vi "FormCalibra7.vi"() -> ()   [LabVIEW 2014]
uses:
  testMachine.ctl
  mainMachine.ctl
  <vilib>/Analysis/baseanly.llb/Mean (DBL).vi
  <vilib>/express/express shared/transition.llb/Dynamic To Waveform Array.vi
  <vilib>/express/express signal manip/GetorSetDDTAttributes/Set DDT Attributes/SetT0.vi
  <vilib>/express/express shared/transition.llb/Waveform Array To Dynamic.vi
  <vilib>/measure/mamon.llb/Trigger Detection for 1 Channel.vi
  <vilib>/express/express signal manip/GetorSetDDTAttributes/Set DDT Attributes/Set DDT Properties.xnode
  <vilib>/Analysis/NI_AALBase.lvlib
  <resource>/objmgr/daqmx.rc
  <vilib>/measure/NI_MAPro.lvlib
panel:
  out "editDistance":dbl caption="Distancia (m)" format="%#_4f"
  in  "Lower level":dbl
  in  "hysteresis":dbl format="%.2p"
  in  "level":dbl format="%.2p"
  out "rpm":bool
  out "deviceName":tag
  out "editTotalWaitLimit":u8
  out "editCountWaitLimit":u8
  out "ledWaitState":bool caption="Wait State"
  out "sliderWaitUpperTime":u8(slide) max=50 scale=0.0..30.0
  out "slideWaitLowerTime":u8(slide) max=30 scale=0.0..1.0
  out "slideWaitTime":u8(slide) scale=0.0..150.0
  out "labelTestTime":string caption="Tempo total de ensaio"
  in  "buttonAcquisition":bool
  in  "editSetWaitTime":u8 caption="Tempo entre ciclos (s)" step=1 format="%0d"
  in  "stop":bool
  out "error out":errorcluster
  out "ledAcquireState":bool caption="Acquire State"
  out "editTotalLowerLimit":u8
  out "editCountLowerLimit":u8
  out "editTotalUpperLimit":u8
  out "editCountUpperLimit":u8
  out "ledEnsaio 3":bool
  out "ledBrakeState":bool caption="Brake State"
  out "ledExitState":bool caption="Exit State"
  out "ledMotorState":bool caption="Motor State"
  out "ledInit2State":bool caption="Init State"
  out "ledBlockState":bool caption="Block State"
  out "ledRunningState":bool caption="Running State"
  out "ledReadyState":bool caption="Ready State"
  out "ledInitState":bool caption="Init State"
  out "mainMachine":T1
  out "testMachine":T2=enum."finish"
  in  "editSetPathToFile":path
  in  "buttonStop":bool
  in  "buttonStart":bool
  out "graphForce":dynamicdata(graph)
  in  "editOffsetForce":dbl caption="Tara" min=0.0 max=100.0 step=0.1
  in  "editSetForce":dbl caption="Fator de conversão"
  out "editForce":dbl caption="Força (Kgf)" format="%#_4f"
  out "graphSpeed":dynamicdata(graph)
  in  "editSetSpeed":dbl caption="Fator de conversão"
  out "editSpeed":dbl caption="Velocidade (km/h)" format="%#_4f"
  out "editEngineSpeed":dbl caption="Rotação (RPM)" format="%#_4f"
  in  "buttonMotor":bool
  in  "buttonBrake":bool
  in  "editSetWaitLowerTime":u8 caption="Tempo de espera (s)"
  in  "editSetWaitUpperTime":u8=3 caption="Tempo de espera (s)"
  in  "editSetNumberOfCycles":u16 caption="Número de ciclos" max=999 step=1 format="%0d"
  in  "editSetLowerLimit":u32 caption="Limite inferior (km/h)"
  in  "editSetUpperLimit":u32 caption="Limite superior (km/h)"
  out "editTempB":dbl caption="Temperatura B (ºC)"
  out "editTempA":dbl caption="Temperatura A (ºC)"
  in  "editSetTempRef":dbl caption="Offset referência" step=0.01 format="%#_2f"
  out "editTempRef":dbl caption="Referência (ºC)"
  out "ledMotor":bool
  out "ledBrake":bool
  out "ledEnsaio":bool
  out "labelTotalCycle":string
  out "labelCurrentCycle":string
  out "labelSystemTitle":string
  in  "editCurrCycleCtr":u32
  in  "velocidade 2":u32
  out "velocidade":u32
  # "Bancada de Frenagem - Ensaio"
  # "Ensaio"
  # "Temperatura"
  # "Rotação"
  # "Célula de Carga"
  # "Configurações do ensaio"
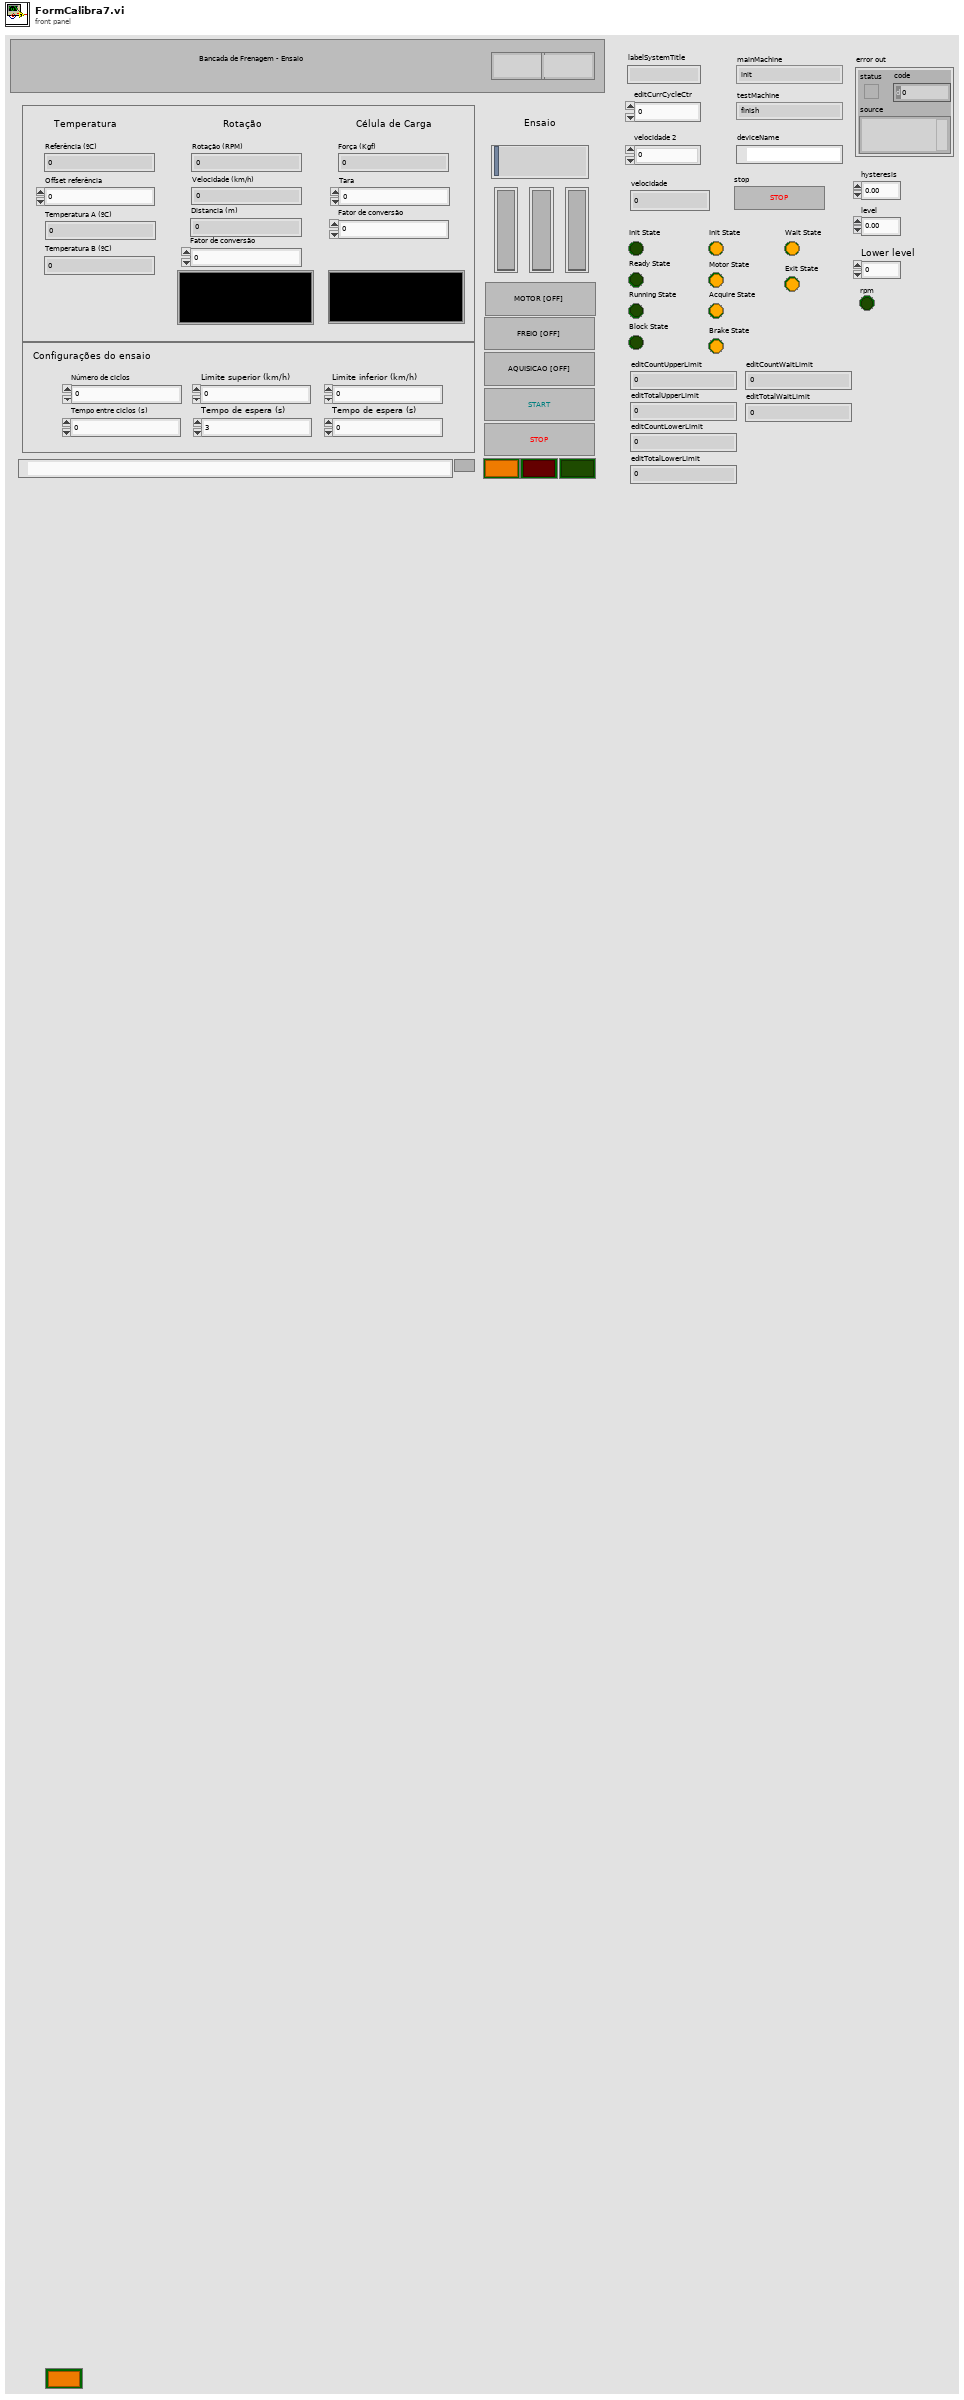
[diagram p1: front panel]
types:
  T1 = typedef "mainMachine.ctl" = enum16{"init", "ready", "running", "blocked", "finish"}
  T2 = typedef "testMachine.ctl" = enum16{"init", "motor", "motor acquire", "brake", "brake acquire", "wait ", "finish", "exit"}
  T3 = enum8{"Enabled", "Disabled", "Disabled and Grayed Out"}
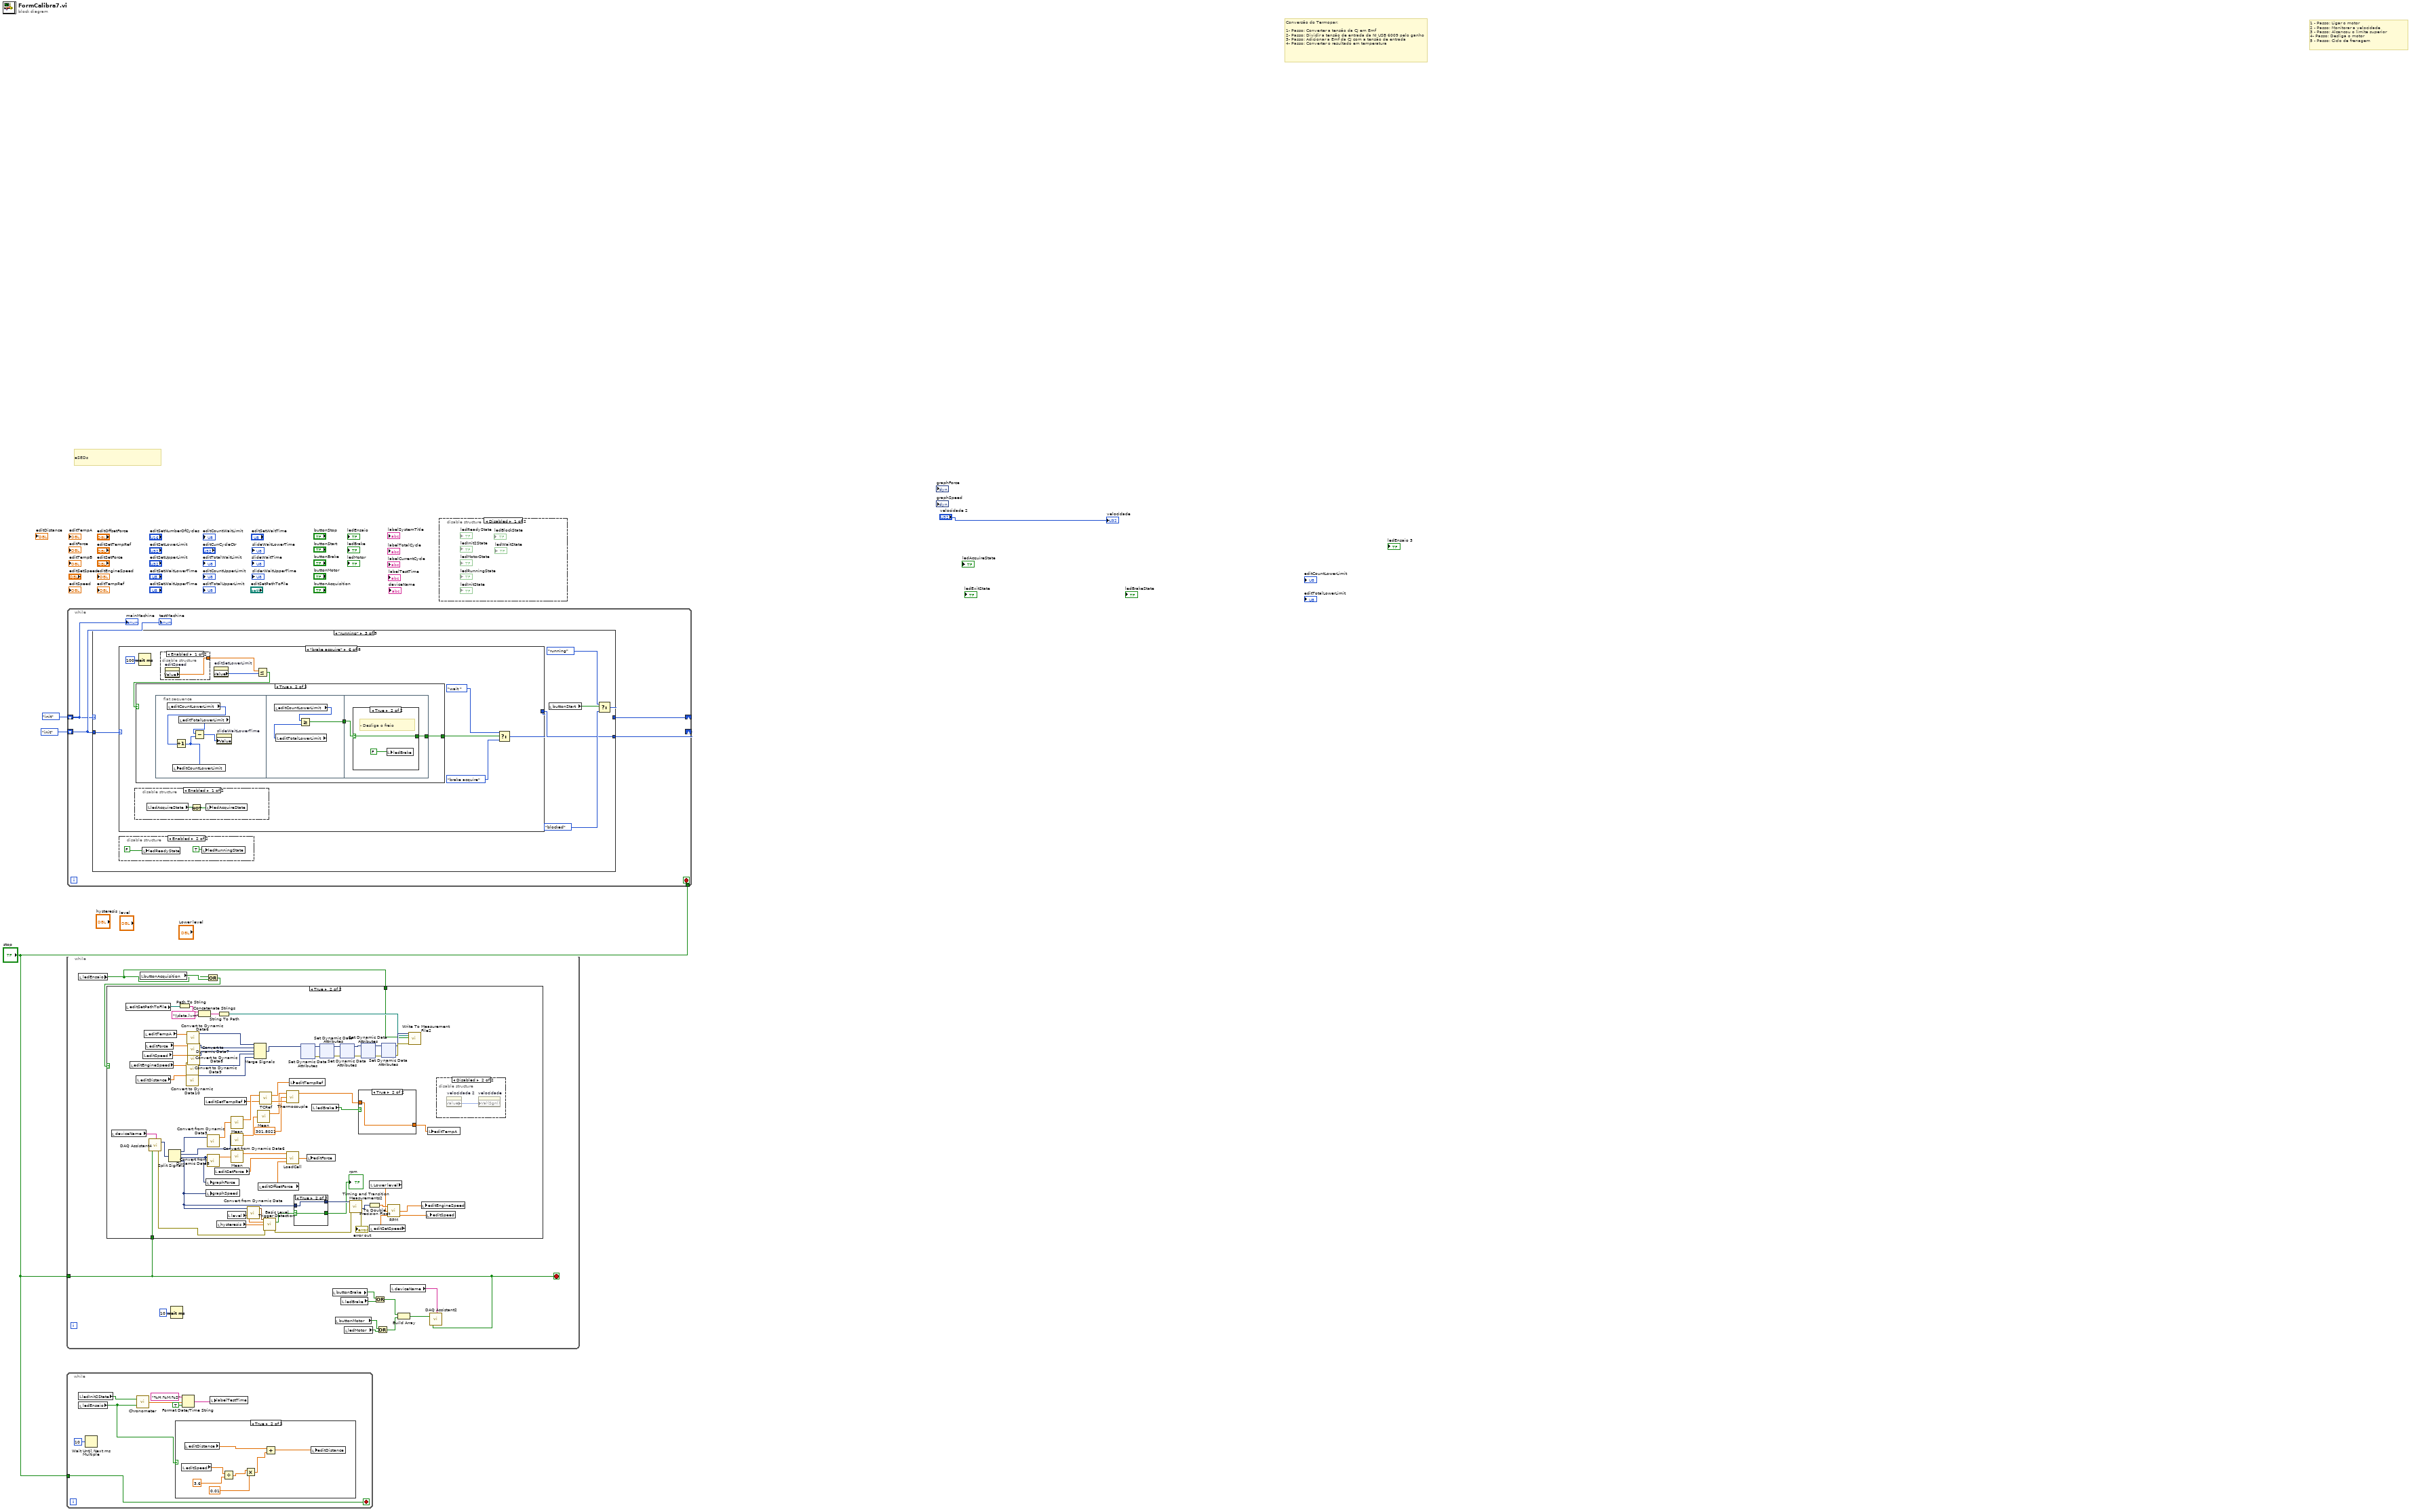
[diagram p0: block diagram]
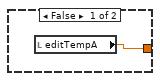
[diagram p5: hidden frame]
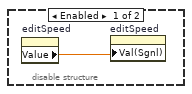
[diagram p7: hidden frame]
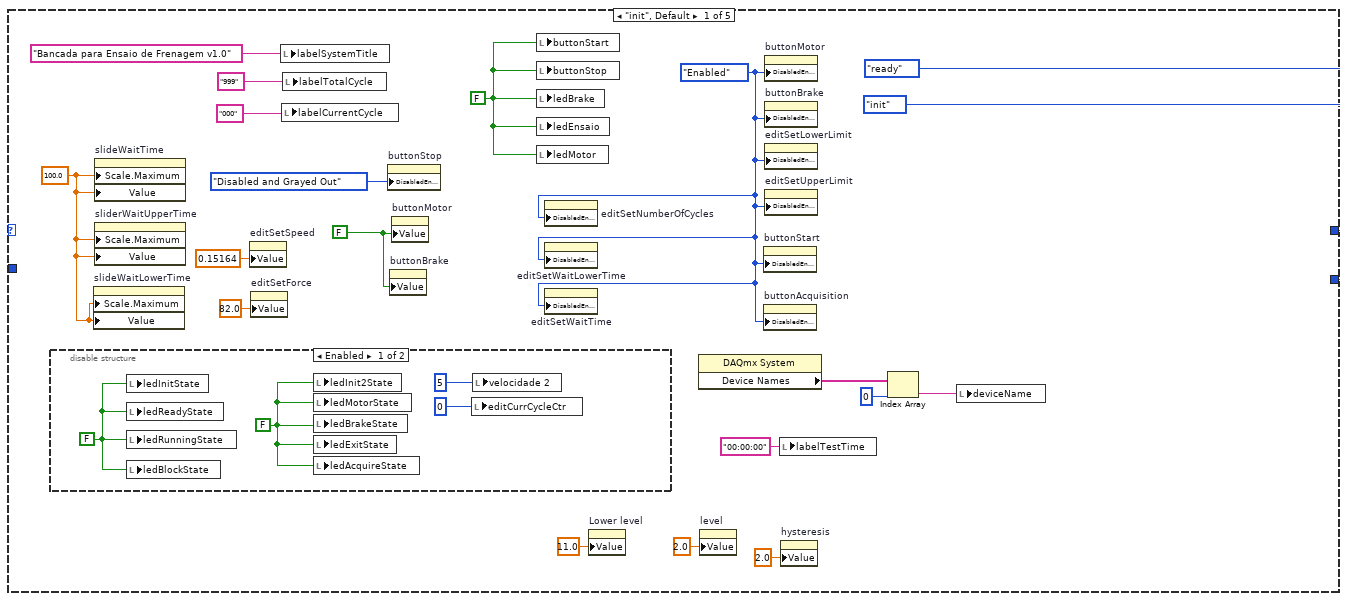
[diagram p8: hidden frame]
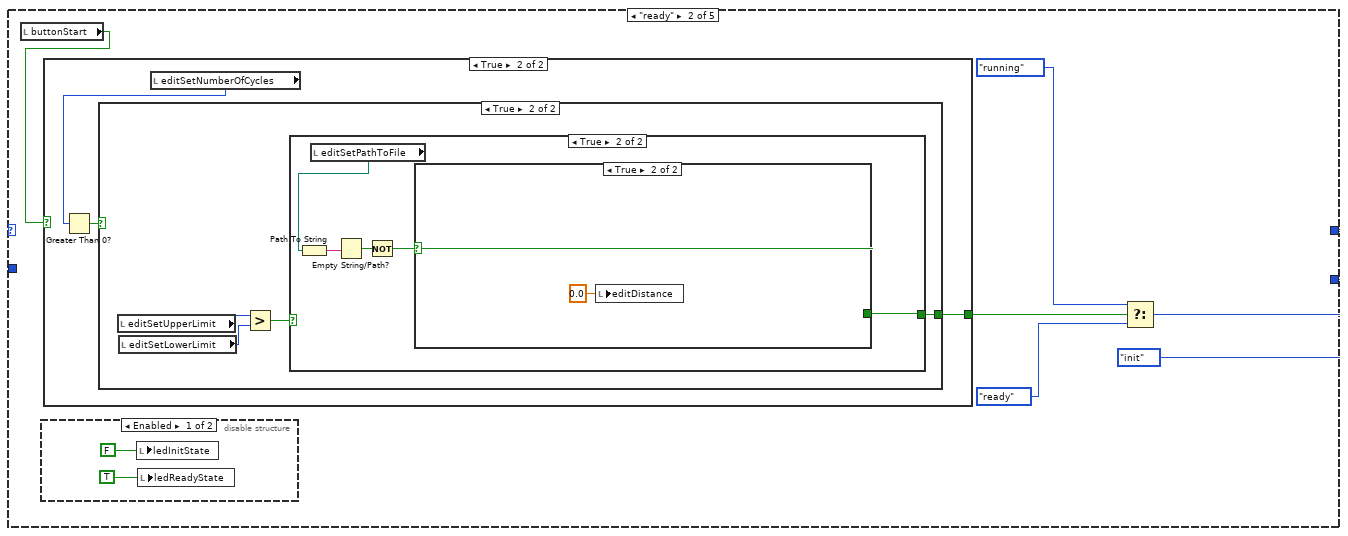
[diagram p10: hidden frame]
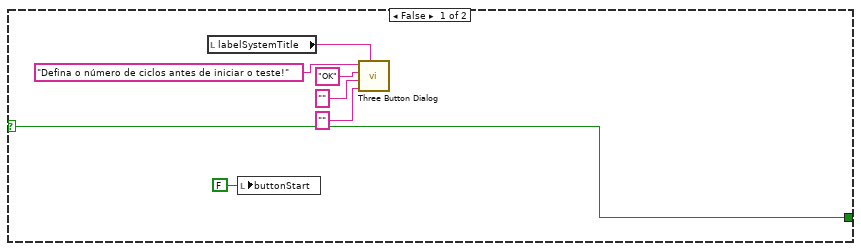
[diagram p13: hidden frame]
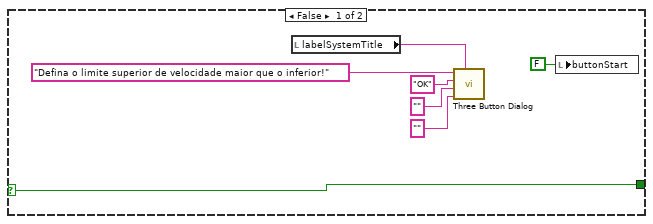
[diagram p14: hidden frame]
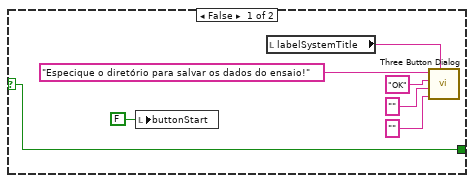
[diagram p15: hidden frame]
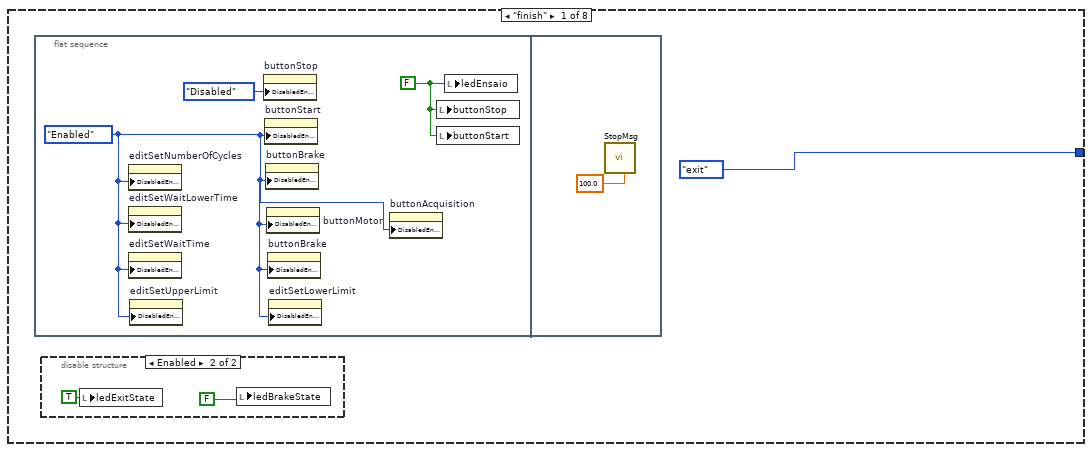
[diagram p17: hidden frame]
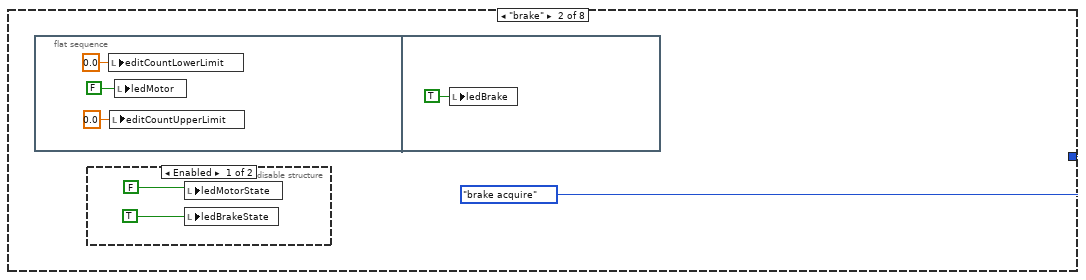
[diagram p19: hidden frame]
diagram:
  # "eSEDs"
  # "1 - Passo: Ligar o motor\n2 - Passo: Monitorar a velocidade\n3 - Passo: Alcancou o limite superior\n4- Passo: Desliga o motor\n5 - Passo: Ciclo de frenagem"
  # "Conversão do Termopar:\n\n1- Passo: Converter a tensão da CJ em Emf\n2- Passo: Dividir a tensão de entrada da NI USB 6009 pelo ganho\n3- Passo: Adicionar a Emf da CJ com a tensão de entrada\n4- Passo: Converter o resultado em temperatura"
  n1 = while {
    tunnel: "stop" -> [w12]
    stop <- w12 stop-if-true
    n2 = local read "ledInit2State"() -> (w7:bool)
    n3 = local read "ledEnsaio"() -> (w5:bool)
    n4 = Wait Until Next ms Multiple(millisecond multiple=u32 10) -> ()  [unwired: 1 out]
    n5 = call "Chronometer.vi"("start"=w5, "reset"=w7) -> ("Time"=w11:dbl)
    n6 = case shown="True" w5 {
      frame False {
      }
      frame True {
        n7 = local read "editSpeed"() -> (w17:dbl)
        n8 = local read "editDistance"() -> (w19:dbl)
        n9 = Divide(x=w17, y=3.6) -> (x/y=w15:dbl)
        n10 = Multiply(x=w15, y=0.01) -> (x*y=w14:dbl)
        n11 = Add(x=w19, y=w14) -> (x+y=w13:dbl)
        n12 = local write "editDistance"(w13) -> ()
      }
    }
    n13 = Format Date/Time String(time format string (%c)="%H:%M:%S", seconds (now)=w11, UTC format=TRUE) -> (date/time string=w8:string)
    n14 = local write "labelTestTime"(w8) -> ()
  }
  n15 = while {
    tunnel: "stop" -> [w25]
    stop <- w25 stop-if-true
    n16 = local read "ledEnsaio"() -> (w22:bool)
    n17 = local read "buttonAcquisition"() -> (w24:bool)
    n18 = Wait (ms)(milliseconds to wait=u32 10) -> ()  [unwired: 1 out]
    n19 = Or(x=w22, y=w24) -> (x .or. y?=w23:bool)
    n20 = case shown="True" w23 {
      tunnel: w25 -> [_ w57]
      tunnel: w22 -> [_ w56]
      frame False {
      }
      frame True {
        n21 = local read "deviceName"() -> (w55:tag)
        n22 = local read "editSetPathToFile"() -> (w77:path)
        n23 = local read "editEngineSpeed"() -> (w39:dbl)
        n24 = local read "editDistance"() -> (w40:dbl)
        n25 = local read "editSpeed"() -> (w37:dbl)
        n26 = local read "editTempA"() -> (w89:dbl)
        n27 = local read "editForce"() -> (w38:dbl)
        n28 = call "DAQ Assistant4"("stop (F)"=w57, "device name"=w55) -> ("data"=w59:dynamicdata, "error out"=w54:errorcluster)  [unwired: 14 in, 2 out]
        n29 = Split Signals(w59) -> (w36:dynamicdata, w35:dynamicdata, w34:dynamicdata, w33:dynamicdata)  [unwired: 4 in]
        n30 = Path To String(path=w77) -> (string=w76:string)
        n31 = call "Convert to Dynamic Data9"("Double"=w39) -> ("Dynamic Data Type"=w93:dynamicdata)  [unwired: 3 in]
        n32 = call "Convert to Dynamic Data10"("Double"=w40) -> ("Dynamic Data Type"=w94:dynamicdata)  [unwired: 3 in]
        n33 = call "Convert to Dynamic Data6"("Double"=w89) -> ("Dynamic Data Type"=w90:dynamicdata)  [unwired: 3 in]
        n34 = call "Convert to Dynamic Data7"("Double"=w38) -> ("Dynamic Data Type"=w91:dynamicdata)  [unwired: 3 in]
        n35 = call "Convert to Dynamic Data8"("Double"=w37) -> ("Dynamic Data Type"=w92:dynamicdata)  [unwired: 3 in]
        n36 = Concatenate Strings(w76, "\\data.lvm" ("string")) -> (w79:string)
        n37 = local read "editSetTempRef"() -> (w61:dbl)
        n38 = local write "graphForce"(w34) -> ()
        n39 = local write "graphSpeed"(w33) -> ()
        n40 = call "Convert from Dynamic Data5"("Dynamic Data Type"=w36) -> ("Array"=w74:dbl[])  [unwired: 3 in]
        n41 = call "Convert from Dynamic Data8"("Dynamic Data Type"=w34) -> ("Array"=w63:dbl[])  [unwired: 3 in]
        n42 = local read "editSetForce"() -> (w72:dbl)
        n43 = local read "hysteresis"() -> (w46:dbl)
        n44 = String To Path(string=w79) -> (path=w80:path)
        n45 = local read "level"() -> (w45:dbl)
        n46 = call-poly <vilib>:"Mean.vi"("X"=w74) -> ("mean"=w75:dbl)  [unwired: 1 out]
        n47 = call "Convert from Dynamic Data6"("Dynamic Data Type"=w35) -> ("Array"=w62:dbl[])  [unwired: 3 in]
        n48 = call-poly <vilib>:"Mean.vi"("X"=w63) -> ("mean"=w67:dbl)  [unwired: 1 out]
        n49 = call "Convert from Dynamic Data"("Dynamic Data Type"=w33) -> ("Waveform"=w51:waveform(dbl))  [unwired: 3 in]
        n50 = Merge Signals(w90, w91, w92, w93, w94) -> (w95:dynamicdata)
        n51 = call-poly <vilib>:"Mean.vi"("X"=w62) -> ("mean"=w64:dbl)  [unwired: 1 out]
        n52 = local read "editOffsetForce"() -> (w73:dbl)
        n53 = call "TCRef.vi"("offset"=w61, "data"=w75) -> ("emf(mV)"=w66:dbl, "temp (degC)"=w60:dbl)
        n54 = call-poly <vilib>:"Basic Level Trigger Detection.vi"("signal in"=w51, "level"=w45, "hysteresis"=w46, "error in (no error)"=w54) -> ("trigger detected?"=w50:bool, "error out"=w53:errorcluster)  [unwired: 9 in, 1 out]
        n55 = call "Thermocouple.vi"("cj(mV)"=w66, "factor"=301.8021, "data"=w64) -> ("temp(degC)"=w42:dbl)  [unwired: 2 out]
        n56 = call "LoadCell.vi"("tara"=w73, "factor"=w72, "data"=w67) -> ("force (Kgf)"=w69:dbl)
        n57 = local write "editTempRef"(w60) -> ()
        n58 = case shown="True" w50 {
          selector: w50 -> [w100 w101]
          tunnel: w33 -> [_ w102]
          tunnel: [_ w102] -> w52
          tunnel: [w100 w101] -> w49
          frame False {
          }
          frame True {
          }
        }
        "rpm" <- w49
        n59 = xnode ("Set Dynamic Data Attributes")("Signals In"=w95) -> ("Signals Out"=w81:dynamicdata, "error out"=w83:errorcluster)  [unwired: 4 in]
        n60 = local write "editForce"(w69) -> ()
        n61 = local read "ledBrake"() -> (w43:bool)
        n62 = xnode ("Set Dynamic Data Attributes")("Signals In"=w81, "error in"=w83) -> ("Signals Out"=w82:dynamicdata, "error out"=w84:errorcluster)  [unwired: 3 in]
        n63 = xnode ("Set Dynamic Data Attributes")("Signals In"=w82, "error in"=w84) -> ("Signals Out"=w96:dynamicdata, "error out"=w85:errorcluster)  [unwired: 3 in]
        n64 = call "Timing and Transition Measurements2"("error in (no error)"=w53, "Signals"=w52) -> ("error out"=→"error out":errorcluster, "Frequency"=w48:dynamicdata)  [unwired: 8 in]
        n65 = case shown="True" w43 {
          tunnel: w42 -> [_ w99]
          tunnel: [w98 w99] -> w41
          frame False {
            n66 = local read "editTempA"() -> (w98:dbl)
          }
          frame True {
          }
        }
        n67 = xnode ("Set Dynamic Data Attributes")("Signals In"=w96, "error in"=w85) -> ("Signals Out"=w97:dynamicdata, "error out"=w86:errorcluster)  [unwired: 3 in]
        n68 = To Double Precision Float(number=w48) -> (double precision float=w47:dbl)
        n69 = local read "Lower level"() -> (w44:dbl)
        n70 = local read "editSetSpeed"() -> (w68:dbl)
        n71 = xnode ("Set Dynamic Data Attributes")("Signals In"=w97, "error in"=w86) -> ("Signals Out"=w87:dynamicdata, "error out"=w88:errorcluster)  [unwired: 3 in]
        n72 = call "RPM.vi"("factor"=w68, "Lower level"=w44, "data"=w47) -> ("km/h"=w71:dbl, "RPM"=w70:dbl)  [unwired: 1 out]
        n73 = call "Write To Measurement File2"("Signals"=w87, "Enable"=w56, "error in (no error)"=w88, "Filename"=w80) -> ()  [unwired: 13 in, 3 out]
        n74 = local write "editEngineSpeed"(w70) -> ()
        n75 = local write "editSpeed"(w71) -> ()
        n76 = local write "editTempA"(w41) -> ()
        n77 = disable-structure shown="Disabled" {
          frame Enabled {
            n78 = property on="editSpeed" class="DigNum (strict)"() -> ("Value"=w103:dbl)  [unwired: 2 in, 2 out]
            n79 = property on="editSpeed" class="DigNum (strict)"("Val(Sgnl)"=w103) -> ()  [unwired: 2 in, 2 out]
          }
          frame Disabled {
            n80 = property on="velocidade 2" class="DigNum (strict)"() -> ("Value"=w104:u32)  [unwired: 2 in, 2 out]
            n81 = property on="velocidade" class="DigNum (strict)"("Val(Sgnl)"=w104) -> ()  [unwired: 2 in, 2 out]
          }
        }
      }
    }
    n82 = local read "buttonBrake"() -> (w29:bool)
    n83 = local read "buttonMotor"() -> (w27:bool)
    n84 = local read "ledBrake"() -> (w31:bool)
    n85 = local read "ledMotor"() -> (w28:bool)
    n86 = Or(x=w29, y=w31) -> (x .or. y?=w30:bool)
    n87 = Or(x=w27, y=w28) -> (x .or. y?=w26:bool)
    n88 = local read "deviceName"() -> (w20:tag)
    n89 = Build Array(w30, w26) -> (w32:bool[])
    n90 = call "DAQ Assistant2"("data"=w32, "stop (T)"=w25, "device name"=w20) -> ()  [unwired: 15 in, 2 out]
  }
  n91 = while {
    shift-right: [w199] -> _
    shift-left: mainMachine."init" ("mainMachine") -> [w196]
    shift-right: [w198] -> _
    shift-left: testMachine."init" ("testMachine") -> [w197]
    tunnel: "stop" -> [w195]
    stop <- w195 stop-if-true
    n92 = case shown="\"running\"" w196 {
      tunnel: [mainMachine."ready" ("mainMachine") w223 w269 w409 mainMachine."finish" ("mainMachine")] -> w199
      tunnel: [testMachine."init" ("testMachine") testMachine."init" ("testMachine") w268 testMachine."init" ("testMachine") testMachine."init" ("testMachine")] -> w198
      tunnel: w197 -> [_ _ w267 _ _]
      frame "init", Default {
        w209 = 100.0 ("Scale.Range:Maximum")
        w210 = T3."Enabled" ("Disabled")
        w211 = FALSE ("buttonMotor")
        w217 = FALSE ("motor")
        n93 = disable-structure shown="Enabled" {
          frame Enabled {
            w219 = FALSE
            w220 = FALSE
            n94 = local write "ledInitState"(w220) -> ()
            n95 = local write "ledReadyState"(w220) -> ()
            n96 = local write "ledRunningState"(w220) -> ()
            n97 = local write "ledBlockState"(w220) -> ()
            n98 = local write "ledInit2State"(w219) -> ()
            n99 = local write "ledMotorState"(w219) -> ()
            n100 = local write "ledBrakeState"(w219) -> ()
            n101 = local write "ledExitState"(w219) -> ()
            n102 = local write "ledAcquireState"(w219) -> ()
            n103 = local write "editCurrCycleCtr"(u32 0 ("currentCycleCtr")) -> ()
            n104 = local write "velocidade 2"(u32 5 ("velocidade 2")) -> ()
          }
          frame Disabled {
          }
        }
        n105 = property on="slideWaitLowerTime" class="Slide (strict)"("Scale.Maximum"=w209, "Value"=w209) -> ()  [unwired: 2 in, 2 out]
        n106 = property on="slideWaitTime" class="Slide (strict)"("Scale.Maximum"=w209, "Value"=w209) -> ()  [unwired: 2 in, 2 out]
        n107 = property on="sliderWaitUpperTime" class="Slide (strict)"("Scale.Maximum"=w209, "Value"=w209) -> ()  [unwired: 2 in, 2 out]
        n108 = property on="editSetSpeed" class="DigNum (strict)"("Value"=0.15164 ("editSetSpeed")) -> ()  [unwired: 2 in, 2 out]
        n109 = property on="editSetForce" class="DigNum (strict)"("Value"=82.0 ("editSetForce")) -> ()  [unwired: 2 in, 2 out]
        n110 = local write "labelSystemTitle"("Bancada para Ensaio de Frenagem v1.0" ("systemTitle")) -> ()
        n111 = local write "labelCurrentCycle"("000" ("currentCycle")) -> ()
        n112 = local write "labelTotalCycle"("999" ("totalCycle")) -> ()
        n113 = property on="buttonStop" class="Bool (strict)"("DisabledEnum"=T3."Disabled and Grayed Out" ("Disabled")) -> ()  [unwired: 2 in, 2 out]
        n114 = property on="buttonBrake" class="Bool (strict)"("Value"=w211) -> ()  [unwired: 2 in, 2 out]
        n115 = property on="buttonMotor" class="Bool (strict)"("Value"=w211) -> ()  [unwired: 2 in, 2 out]
        n116 = local write "buttonStart"(w217) -> ()
        n117 = local write "buttonStop"(w217) -> ()
        n118 = local write "ledBrake"(w217) -> ()
        n119 = local write "ledEnsaio"(w217) -> ()
        n120 = local write "ledMotor"(w217) -> ()
        n121 = property on="editSetNumberOfCycles" class="DigNum (strict)"("DisabledEnum"=w210) -> ()  [unwired: 2 in, 2 out]
        n122 = property on="editSetWaitLowerTime" class="DigNum (strict)"("DisabledEnum"=w210) -> ()  [unwired: 2 in, 2 out]
        n123 = property on="editSetWaitTime" class="DigNum (strict)"("DisabledEnum"=w210) -> ()  [unwired: 2 in, 2 out]
        n124 = property on="Lower level" class="DigNum (strict)"("Value"=11.0 ("Lower level")) -> ()  [unwired: 2 in, 2 out]
        n125 = property class="DAQmx System"() -> ("Device Names"=w208:tag[])  [unwired: 2 in, 2 out]
        n126 = property on="level" class="DigNum (strict)"("Value"=2.0 ("level")) -> ()  [unwired: 2 in, 2 out]
        n127 = property on="buttonStart" class="Bool (strict)"("DisabledEnum"=w210) -> ()  [unwired: 2 in, 2 out]
        n128 = property on="buttonAcquisition" class="Bool (strict)"("DisabledEnum"=w210) -> ()  [unwired: 2 in, 2 out]
        n129 = property on="buttonMotor" class="Bool (strict)"("DisabledEnum"=w210) -> ()  [unwired: 2 in, 2 out]
        n130 = property on="buttonBrake" class="Bool (strict)"("DisabledEnum"=w210) -> ()  [unwired: 2 in, 2 out]
        n131 = property on="editSetLowerLimit" class="DigNum (strict)"("DisabledEnum"=w210) -> ()  [unwired: 2 in, 2 out]
        n132 = property on="editSetUpperLimit" class="DigNum (strict)"("DisabledEnum"=w210) -> ()  [unwired: 2 in, 2 out]
        n133 = local write "labelTestTime"("00:00:00" ("labelTestTime")) -> ()
        n134 = property on="hysteresis" class="DigNum (strict)"("Value"=2.0 ("hysteresis")) -> ()  [unwired: 2 in, 2 out]
        n135 = Index Array(array=w208, index=0) -> (element=w206:tag)
        n136 = local write "deviceName"(w206) -> ()
      }
      frame "ready" {
        n137 = local read "buttonStart"() -> (w226:bool)
        n138 = disable-structure shown="Enabled" {
          frame Enabled {
            n139 = local write "ledInitState"(FALSE ("ledReady")) -> ()
            n140 = local write "ledReadyState"(TRUE ("ledReady")) -> ()
          }
          frame Disabled {
          }
        }
        n141 = case shown="True" w226 {
          selector: w226 -> [w231 _]
          tunnel: [w231 w232] -> w225
          frame False {
          }
          frame True {
            n142 = local read "editSetNumberOfCycles"() -> (w233:u16)
            n143 = Greater Than 0?(x=w233) -> (x > 0?=w234:bool)
            n144 = case shown="True" w234 {
              selector: w234 -> [w241 _]
              tunnel: [w241 w242] -> w232
              frame False {
                n145 = local read "labelSystemTitle"() -> (w236:string)
                n146 = local write "buttonStart"(FALSE ("startButton")) -> ()
                n147 = call <vilib>:"Three Button Dialog.vi"("Window Title (\"\")"=w236, "Right Button Text (\"Cancel\")"="" ("Right Button Text (\"Cancel\")"), "Center Button Text (\"No\")"="" ("Center Button Text (\"No\")"), "Left Button Text (\"Yes\")"="OK" ("Left Button Text (\"Yes\")"), "message"="Defina o número de ciclos antes de iniciar o teste!") -> ()  [unwired: 6 in, 1 out]
              }
              frame True {
                n148 = local read "editSetUpperLimit"() -> (w244:u32)
                n149 = local read "editSetLowerLimit"() -> (w243:u32)
                n150 = Greater?(x=w244, y=w243) -> (0:w245:bool)
                n151 = case shown="True" w245 {
                  selector: w245 -> [w252 _]
                  tunnel: [w252 w255] -> w242
                  frame False {
                    n152 = local read "labelSystemTitle"() -> (w247:string)
                    n153 = call <vilib>:"Three Button Dialog.vi"("Window Title (\"\")"=w247, "Right Button Text (\"Cancel\")"="" ("Right Button Text (\"Cancel\")"), "Center Button Text (\"No\")"="" ("Center Button Text (\"No\")"), "Left Button Text (\"Yes\")"="OK" ("Left Button Text (\"Yes\")"), "message"="Defina o limite superior de velocidade maior que o inferior!") -> ()  [unwired: 6 in, 1 out]
                    n154 = local write "buttonStart"(FALSE ("startButton")) -> ()
                  }
                  frame True {
                    n155 = local read "editSetPathToFile"() -> (w257:path)
                    n156 = Path To String(path=w257) -> (string=w256:string)
                    n157 = Empty String/Path?(string/path=w256) -> (empty?=w254:bool)
                    n158 = Not(x=w254) -> (.not. x?=w253:bool)
                    n159 = case shown="True" w253 {
                      selector: w253 -> [w264 w266]
                      tunnel: [w264 w266] -> w255
                      frame False {
                        n160 = local write "buttonStart"(FALSE ("startButton")) -> ()
                        n161 = local read "labelSystemTitle"() -> (w259:string)
                        n162 = call <vilib>:"Three Button Dialog.vi"("Window Title (\"\")"=w259, "Right Button Text (\"Cancel\")"="" ("Right Button Text (\"Cancel\")"), "Center Button Text (\"No\")"="" ("Center Button Text (\"No\")"), "Left Button Text (\"Yes\")"="OK" ("Left Button Text (\"Yes\")"), "message"="Especique o diretório para salvar os dados do ensaio!") -> ()  [unwired: 6 in, 1 out]
                      }
                      frame True {
                        n163 = local write "editDistance"(0.0 ("editDistance")) -> ()
                      }
                    }
                  }
                }
              }
            }
          }
        }
        n164 = Select(t=mainMachine."running" ("mainMachine"), s=w225, f=mainMachine."ready" ("mainMachine")) -> (s? t:f=w223:T1)
      }
      frame "running" {
        n165 = case shown="\"brake acquire\"" w267 {
          tunnel: [testMachine."exit" ("testMachine") testMachine."brake acquire" ("testMachine") testMachine."motor acquire" ("testMachine") testMachine."motor" ("testMachine") w339 w359 testMachine."exit" ("testMachine") w392] -> w268
          frame "finish" {
            n166 = flat-sequence {
              frame #0 {
                w279 = FALSE ("ledReady")
                w278 = T3."Enabled" ("Disabled")
                n167 = property on="editSetNumberOfCycles" class="DigNum (strict)"("DisabledEnum"=w278) -> ()  [unwired: 2 in, 2 out]
                n168 = property on="editSetWaitLowerTime" class="DigNum (strict)"("DisabledEnum"=w278) -> ()  [unwired: 2 in, 2 out]
                n169 = property on="editSetWaitTime" class="DigNum (strict)"("DisabledEnum"=w278) -> ()  [unwired: 2 in, 2 out]
                n170 = property on="editSetUpperLimit" class="DigNum (strict)"("DisabledEnum"=w278) -> ()  [unwired: 2 in, 2 out]
                n171 = property on="buttonStop" class="Bool (strict)"("DisabledEnum"=T3."Disabled" ("Disabled")) -> ()  [unwired: 2 in, 2 out]
                n172 = property on="buttonStart" class="Bool (strict)"("DisabledEnum"=w278) -> ()  [unwired: 2 in, 2 out]
                n173 = property on="buttonBrake" class="Bool (strict)"("DisabledEnum"=w278) -> ()  [unwired: 2 in, 2 out]
                n174 = property on="buttonMotor" class="Bool (strict)"("DisabledEnum"=w278) -> ()  [unwired: 2 in, 2 out]
                n175 = property on="buttonBrake" class="Bool (strict)"("DisabledEnum"=w278) -> ()  [unwired: 2 in, 2 out]
                n176 = property on="editSetLowerLimit" class="DigNum (strict)"("DisabledEnum"=w278) -> ()  [unwired: 2 in, 2 out]
                n177 = property on="buttonAcquisition" class="Bool (strict)"("DisabledEnum"=w278) -> ()  [unwired: 2 in, 2 out]
                n178 = local write "buttonStop"(w279) -> ()
                n179 = local write "buttonStart"(w279) -> ()
                n180 = local write "ledEnsaio"(w279) -> ()
              }
              frame #1 {
                n181 = call "StopMsg.vi"("Max Value (100)"=100.0) -> ()  [unwired: 8 in, 2 out]
              }
            }
            n182 = disable-structure shown="Enabled" {
              frame Disabled {
              }
              frame Enabled {
                n183 = local write "ledExitState"(TRUE ("ledReady")) -> ()
                n184 = local write "ledBrakeState"(FALSE ("ledReady")) -> ()
              }
            }
          }
          frame "brake" {
            n185 = flat-sequence {
              frame #0 {
                n186 = local write "editCountLowerLimit"(0.0 ("editCountUpperLimit")) -> ()
                n187 = local write "editCountUpperLimit"(0.0 ("editCountUpperLimit")) -> ()
                n188 = local write "ledMotor"(FALSE ("motor")) -> ()
              }
              frame #1 {
                n189 = local write "ledBrake"(TRUE ("freio")) -> ()
              }
            }
            n190 = disable-structure shown="Enabled" {
              frame Enabled {
                n191 = local write "ledMotorState"(FALSE ("ledReady")) -> ()
                n192 = local write "ledBrakeState"(TRUE ("ledReady")) -> ()
              }
              frame Disabled {
              }
            }
          }
          frame "motor" {
            n193 = flat-sequence {
              frame #0 {
                n194 = local read "editCurrCycleCtr"() -> (w294:u32)
                n195 = Increment(x=w294) -> (x+1=w293:u32)
                n196 = local write "editCurrCycleCtr"(w293) -> ()
              }
              frame #1 {
                n197 = local read "editCurrCycleCtr"() -> (w301:u32)
                n198 = local read "editTotalWaitLimit"() -> (w295:u8)
                n199 = local read "editTotalUpperLimit"() -> (w297:u8)
                n200 = local read "editTotalLowerLimit"() -> (w296:u8)
                n201 = local write "editCountLowerLimit"(u8 0 ("editCountLowerLimit")) -> ()
                n202 = local write "editCountWaitLimit"(u8 0 ("editCountWaitLimit")) -> ()
                n203 = local write "editCountUpperLimit"(u8 0 ("editCountUpperLimit")) -> ()
                n204 = Format Into String(format string="%03d", w301) -> (resulting string=w302:string)  [unwired: 2 in, 1 out]
                n205 = property on="sliderWaitUpperTime" class="Slide (strict)"("Value"=w297) -> ()  [unwired: 2 in, 2 out]
                n206 = property on="slideWaitLowerTime" class="Slide (strict)"("Value"=w296) -> ()  [unwired: 2 in, 2 out]
                n207 = property on="slideWaitTime" class="Slide (strict)"("Value"=w295) -> ()  [unwired: 2 in, 2 out]
                n208 = local write "labelCurrentCycle"(w302) -> ()
              }
              frame #2 {
                # "- Liga o motor"
                n209 = local write "ledMotor"(TRUE ("motor")) -> ()
                n210 = property on="buttonStop" class="Bool (strict)"("DisabledEnum"=T3."Enabled" ("Disabled")) -> ()  [unwired: 2 in, 2 out]
                n211 = property on="buttonStart" class="Bool (strict)"("DisabledEnum"=T3."Disabled and Grayed Out" ("Disabled")) -> ()  [unwired: 2 in, 2 out]
              }
            }
            n212 = disable-structure shown="Enabled" {
              frame Enabled {
                n213 = local write "ledInit2State"(FALSE ("ledReady")) -> ()
                n214 = local write "ledBrakeState"(FALSE ("ledReady")) -> ()
                n215 = local write "ledMotorState"(TRUE ("ledReady")) -> ()
              }
              frame Disabled {
              }
            }
          }
          frame "init", Default {
            n216 = stacked-sequence {
              frame #0 {
                w314 = FALSE ("ensaio")
                n217 = property on="buttonBrake" class="Bool (strict)"("Value"=w314) -> ()  [unwired: 2 in, 2 out]
                n218 = local write "ledMotor"(w314) -> ()
                n219 = local write "ledBrake"(w314) -> ()
                n220 = property on="buttonMotor" class="Bool (strict)"("Value"=w314) -> ()  [unwired: 2 in, 2 out]
                n221 = local read "editSetNumberOfCycles"() -> (w321:u16)
                n222 = local read "editSetWaitLowerTime"() -> (w315:u8)
                n223 = local read "editSetWaitUpperTime"() -> (w318:u8)
                n224 = local read "editSetWaitTime"() -> (w309:u8)
                n225 = Multiply(x=w309, y=u32 10) -> (x*y=w310:u32)
                n226 = Multiply(x=w315, y=u32 10) -> (x*y=w313:u32)
                n227 = Format Into String(format string="%03d", w321) -> (resulting string=w322:string)  [unwired: 2 in, 1 out]
                n228 = Multiply(x=w318, y=u32 10) -> (x*y=w312:u32)
                n229 = local write "editTotalLowerLimit"(w313) -> ()
                n230 = local write "editTotalUpperLimit"(w312) -> ()
                n231 = local write "editTotalWaitLimit"(w310) -> ()
                n232 = local write "labelTotalCycle"(w322) -> ()
                n233 = local write "editCurrCycleCtr"(u32 0 ("currentCycleCtr")) -> ()
                n234 = local write "labelCurrentCycle"("000" ("currentCycle")) -> ()
              }
              frame #1 {
                w330 = T3."Disabled" ("Disabled")
                n235 = property on="editSetNumberOfCycles" class="DigNum (strict)"("DisabledEnum"=w330) -> ()  [unwired: 2 in, 2 out]
                n236 = property on="editSetWaitLowerTime" class="DigNum (strict)"("DisabledEnum"=w330) -> ()  [unwired: 2 in, 2 out]
                n237 = property on="editSetWaitTime" class="DigNum (strict)"("DisabledEnum"=w330) -> ()  [unwired: 2 in, 2 out]
                n238 = local read "editTotalUpperLimit"() -> (w333:u8)
                n239 = property on="sliderWaitUpperTime" class="Slide (strict)"("Scale.Maximum"=w333, "Scale.Minimum"=0.0 ("Scale.Range:Minimum"), "Scale.Increment"=1.0 ("Scale.Range:Increment"), "Value"=w333) -> ()  [unwired: 2 in, 2 out]
                n240 = property on="buttonAcquisition" class="Bool (strict)"("DisabledEnum"=w330) -> ()  [unwired: 2 in, 2 out]
                n241 = local read "editTotalLowerLimit"() -> (w327:u8)
                n242 = property on="slideWaitLowerTime" class="Slide (strict)"("Scale.Maximum"=w327, "Scale.Minimum"=0.0 ("Scale.Range:Minimum"), "Scale.Increment"=1.0 ("Scale.Range:Increment"), "Value"=w327) -> ()  [unwired: 2 in, 2 out]
                n243 = local read "editTotalWaitLimit"() -> (w324:u8)
                n244 = property on="slideWaitTime" class="Slide (strict)"("Scale.Maximum"=w324, "Scale.Minimum"=0.0 ("Scale.Range:Minimum"), "Scale.Increment"=1.0 ("Scale.Range:Increment"), "Value"=w324) -> ()  [unwired: 2 in, 2 out]
                n245 = call "StarMsg.vi"("Show"=TRUE, "Max Value (100)"=100.0) -> ()  [unwired: 7 in, 2 out]
                n246 = property on="buttonMotor" class="Bool (strict)"("DisabledEnum"=w330) -> ()  [unwired: 2 in, 2 out]
                n247 = property on="buttonBrake" class="Bool (strict)"("DisabledEnum"=w330) -> ()  [unwired: 2 in, 2 out]
                n248 = property on="editSetLowerLimit" class="DigNum (strict)"("DisabledEnum"=w330) -> ()  [unwired: 2 in, 2 out]
                n249 = property on="editSetUpperLimit" class="DigNum (strict)"("DisabledEnum"=w330) -> ()  [unwired: 2 in, 2 out]
              }
              frame #2 {
                n250 = local write "ledEnsaio"(TRUE ("ensaio")) -> ()
              }
            }
            n251 = disable-structure shown="Enabled" {
              frame Enabled {
                n252 = local write "ledInit2State"(TRUE ("ledReady")) -> ()
              }
              frame Disabled {
              }
            }
          }
          frame "motor acquire" {
            n253 = disable-structure shown="Enabled" {
              frame Enabled {
                n254 = local read "ledAcquireState"() -> (w348:bool)
                n255 = Not(x=w348) -> (.not. x?=w347:bool)
                n256 = local write "ledAcquireState"(w347) -> ()
              }
              frame Disabled {
              }
            }
            n257 = Wait (ms)(milliseconds to wait=u32 100) -> ()  [unwired: 1 out]
            n258 = disable-structure shown="Enabled" {
              disable-tunnel: [w345 w346] -> w338
              frame Enabled {
                n259 = property on="editSpeed" class="DigNum (strict)"() -> ("Value"=w345:dbl)  [unwired: 2 in, 2 out]
              }
              frame Disabled {
                n260 = property on="velocidade" class="DigNum (strict)"() -> ("Value"=w346:u32)  [unwired: 2 in, 2 out]
              }
            }
            n261 = property on="editSetUpperLimit" class="DigNum (strict)"() -> ("Value"=w337:u32)  [unwired: 2 in, 2 out]
            n262 = Greater Or Equal?(x=w338, y=w337) -> (x >= y?=w343:bool)
            n263 = case shown="True" w343 {
              selector: w343 -> [w349 _]
              tunnel: [w349 w350] -> w342
              frame False {
              }
              frame True {
                n264 = flat-sequence {
                  tunnel: [w355] -> w350
                  frame #0 {
                    n265 = local read "editCountUpperLimit"() -> (w353:u8)
                    n266 = Increment(x=w353) -> (x+1=w351:u8)
                    n267 = local write "editCountUpperLimit"(w351) -> ()
                    n268 = local read "editTotalUpperLimit"() -> (w352:u8)
                    n269 = Subtract(x=w352, y=w351) -> (x-y=w354:u8)
                    n270 = property on="sliderWaitUpperTime" class="Slide (strict)"("Value"=w354) -> ()  [unwired: 2 in, 2 out]
                  }
                  frame #1 {
                    n271 = local read "editCountUpperLimit"() -> (w357:u8)
                    n272 = local read "editTotalUpperLimit"() -> (w356:u8)
                    n273 = Greater Or Equal?(x=w357, y=w356) -> (x >= y?=w355:bool)
                  }
                }
              }
            }
            n274 = Select(t=testMachine."brake" ("testMachine"), s=w342, f=testMachine."motor acquire" ("testMachine")) -> (s? t:f=w339:T2)
          }
          frame "brake acquire" {
            n275 = disable-structure shown="Enabled" {
              frame Enabled {
                n276 = local read "ledAcquireState"() -> (w367:bool)
                n277 = Not(x=w367) -> (.not. x?=w366:bool)
                n278 = local write "ledAcquireState"(w366) -> ()
              }
              frame Disabled {
              }
            }
            n279 = Wait (ms)(milliseconds to wait=u32 100) -> ()  [unwired: 1 out]
            n280 = disable-structure shown="Enabled" {
              disable-tunnel: [w368 w369] -> w358
              frame Enabled {
                n281 = property on="editSpeed" class="DigNum (strict)"() -> ("Value"=w368:dbl)  [unwired: 2 in, 2 out]
              }
              frame Disabled {
                n282 = property on="velocidade" class="DigNum (strict)"() -> ("Value"=w369:u32)  [unwired: 2 in, 2 out]
              }
            }
            n283 = property on="editSetLowerLimit" class="DigNum (strict)"() -> ("Value"=w360:u32)  [unwired: 2 in, 2 out]
            n284 = Less Or Equal?(x=w358, y=w360) -> (x <= y?=w364:bool)
            n285 = case shown="True" w364 {
              selector: w364 -> [w370 _]
              tunnel: [w370 w371] -> w362
              frame False {
              }
              frame True {
                n286 = flat-sequence {
                  tunnel: [w377] -> w372
                  tunnel: w372 -> [w381]
                  tunnel: [w380] -> w371
                  frame #0 {
                    n287 = local read "editCountLowerLimit"() -> (w376:u8)
                    n288 = Increment(x=w376) -> (x+1=w375:u8)
                    n289 = local write "editCountLowerLimit"(w375) -> ()
                    n290 = local read "editTotalLowerLimit"() -> (w374:u8)
                    n291 = Subtract(x=w374, y=w375) -> (x-y=w373:u8)
                    n292 = property on="slideWaitLowerTime" class="Slide (strict)"("Value"=w373) -> ()  [unwired: 2 in, 2 out]
                  }
                  frame #1 {
                    n293 = local read "editCountLowerLimit"() -> (w379:u8)
                    n294 = local read "editTotalLowerLimit"() -> (w378:u8)
                    n295 = Greater Or Equal?(x=w379, y=w378) -> (x >= y?=w377:bool)
                  }
                  frame #2 {
                    n296 = case shown="True" w381 {
                      selector: w381 -> [w382 w383]
                      tunnel: [w382 w383] -> w380
                      frame False {
                      }
                      frame True {
                        # "- Desliga o freio"
                        n297 = local write "ledBrake"(FALSE ("freio")) -> ()
                      }
                    }
                  }
                }
              }
            }
            n298 = Select(t=testMachine."wait " ("testMachine"), s=w362, f=testMachine."brake acquire" ("testMachine")) -> (s? t:f=w359:T2)
          }
          frame "exit" {
          }
          frame "wait " {
            # "- Aguarda 0.5s \n- Atualiza o numero de ciclos"
            n299 = flat-sequence {
              tunnel: [w398] -> w386
              frame #0 {
                n300 = local read "editCountWaitLimit"() -> (w394:u8)
                n301 = Increment(x=w394) -> (x+1=w395:u8)
                n302 = local write "editCountWaitLimit"(w395) -> ()
                n303 = local read "editTotalWaitLimit"() -> (w397:u8)
                n304 = Subtract(x=w397, y=w395) -> (x-y=w396:u8)
                n305 = property on="slideWaitTime" class="Slide (strict)"("Value"=w396) -> ()  [unwired: 2 in, 2 out]
              }
              frame #1 {
                n306 = local read "editCountWaitLimit"() -> (w400:u8)
                n307 = local read "editTotalWaitLimit"() -> (w399:u8)
                n308 = Greater Or Equal?(x=w400, y=w399) -> (x >= y?=w398:bool)
              }
            }
            n309 = disable-structure shown="Enabled" {
              frame Enabled {
                n310 = local read "ledWaitState"() -> (w407:bool)
                n311 = Not(x=w407) -> (.not. x?=w406:bool)
                n312 = local write "ledBrakeState"(FALSE ("ledBrakeState")) -> ()
                n313 = local write "ledWaitState"(w406) -> ()
              }
              frame Disabled {
              }
            }
            n314 = Wait (ms)(milliseconds to wait=u32 100) -> ()  [unwired: 1 out]
            n315 = case shown="True" w386 {
              selector: w386 -> [w401 _]
              tunnel: [w401 w405] -> w387
              frame False {
              }
              frame True {
                n316 = local read "editSetNumberOfCycles"() -> (w403:u16)
                n317 = local read "editCurrCycleCtr"() -> (w402:u32)
                n318 = Greater Or Equal?(x=w402, y=w403) -> (x >= y?=w405:bool)
                n319 = Not(x=w405) -> (.not. x?=w404:bool)
                n320 = local write "ledEnsaio"(w404) -> ()
              }
            }
            n321 = Select(t=testMachine."motor" ("testMachine"), s=w386, f=testMachine."wait " ("testMachine")) -> (s? t:f=w388:T2)
            n322 = Select(t=testMachine."finish" ("testMachine"), s=w387, f=w388) -> (s? t:f=w392:T2)
          }
        }
        n323 = disable-structure shown="Enabled" {
          frame Disabled {
          }
          frame Enabled {
            n324 = local write "ledReadyState"(FALSE ("ledReady")) -> ()
            n325 = local write "ledRunningState"(TRUE ("ledReady")) -> ()
          }
        }
        n326 = local read "buttonStart"() -> (w272:bool)
        n327 = Select(t=mainMachine."running" ("mainMachine"), s=w272, f=mainMachine."blocked" ("mainMachine")) -> (s? t:f=w269:T1)
      }
      frame "blocked" {
        n328 = local read "buttonStart"() -> (w413:bool)
        n329 = Select(t=mainMachine."ready" ("mainMachine"), s=w413, f=mainMachine."blocked" ("mainMachine")) -> (s? t:f=w409:T1)
        n330 = local write "ledRunningState"(FALSE ("ledReady")) -> ()
        n331 = local write "ledBlockState"(TRUE ("ledReady")) -> ()
      }
      frame "finish" {
        n332 = local write "ledBlockState"(FALSE ("ledReady")) -> ()
      }
    }
    "mainMachine" <- w196
    "testMachine" <- w197
  }
  n333 = disable-structure shown="Disabled" {
    frame Disabled {
    }
    frame Enabled {
    }
  }
  "velocidade" <- "velocidade 2"
